vi "Example 2 Primitive Lottery.vi"() -> ()   [LabVIEW 2020]
uses:
  <vilib>/measure/NI_MABase.lvlib
panel:
  out "Fs":dbl format="%#_13g"
  out "Nyquist Eqn":string
  out "cycle of signals":i32
  out "Waveform Graph":waveform(dbl)(graph)
  in  "stop":bool
  in  "amplitude  noise":dbl(knob)=1.0 min=0.001 max=1.0 step=0.1 scale=0.001..1.0
  in  "frequency":dbl(knob)=100.0 min=100.0 max=10000.0 step=10.0 scale=100.0..10000.0
  in  "amplitude":dbl(knob)=1.0 min=0.1 max=10.0 step=0.1 scale=0.1..10.0
  in  "phase":dbl(slide) min=0.0 max=360.0 step=5.0 scale=0.0..360.0
  in  "signal type":T1(ring)
  in  "sampling info":cluster{"Fs":dbl, "#s":dbl}={"Fs"=1000.0, "#s"=1000.0} {"Fs" format="%.2p"}
  in  "square wave duty cycle (%)":dbl=50.0 format="%0.2f"
  in  "offset":dbl(slide)=0.005 min=0.005 max=5.0 step=0.1 scale=0.005..5.0
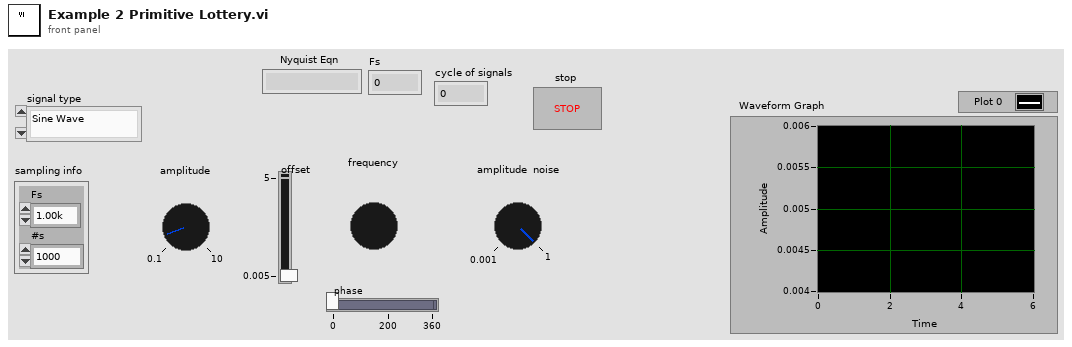
[diagram p1: front panel]
types:
  T1 = enum16{"Sine Wave", "Triangle Wave", "Square Wave", "Sawtooth Wave"}
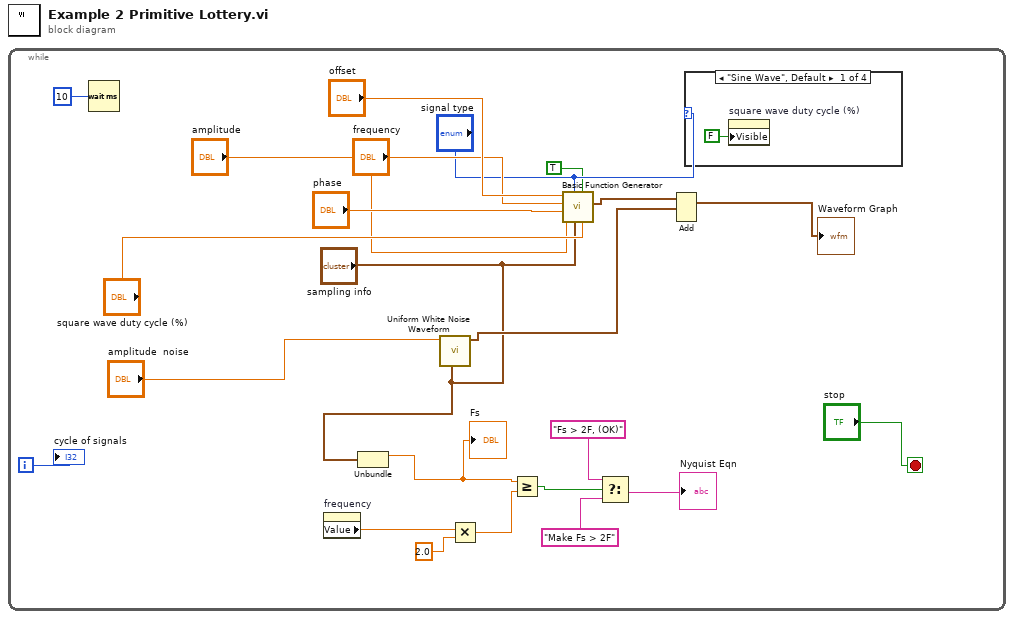
[diagram p0: block diagram]
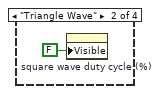
[diagram p2: hidden frame]
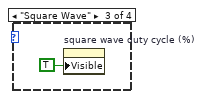
[diagram p3: hidden frame]
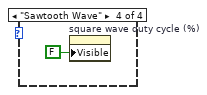
[diagram p4: hidden frame]
diagram:
  n1 = while {
    i -> [w12]
    stop <- "stop" stop-if-true
    n2 = Wait (ms)(milliseconds to wait=10) -> ()  [unwired: 1 out]
    n3 = property on="frequency" class="Knob (strict)"() -> ("Value"=w4:dbl)  [unwired: 2 in, 2 out]
    n4 = Unbundle("sampling info") -> ("Fs"=w2:dbl)  [unwired: 1 out]
    "Fs" <- w2
    n5 = call <vilib>:"Uniform White Noise Waveform.vi"("sampling info"="sampling info", "amplitude"="amplitude  noise") -> ("signal out"=w15:waveform(dbl))  [unwired: 8 in, 1 out]
    n6 = Multiply(x=w4, y=2.0) -> (x*y=w6:dbl)
    n7 = Greater Or Equal?(x=w2, y=w6) -> (x >= y?=w8:bool)
    n8 = call <vilib>:"Basic Function Generator.vi"("offset"="offset", "square wave duty cycle (%)"="square wave duty cycle (%)", "reset signal"=TRUE, "sampling info"="sampling info", "signal type"="signal type", "phase"="phase", "amplitude"="amplitude", "frequency"="frequency") -> ("signal out"=w16:waveform(dbl))  [unwired: 1 in, 2 out]
    n9 = Select(t="Fs > 2F, (OK)", s=w8, f="Make Fs > 2F") -> (s? t:f=→"Nyquist Eqn":string)
    n10 = Add(1:w15, 2:w16) -> (0:→"Waveform Graph":waveform(dbl))  [unwired: 1 in, 1 out]
    n11 = case shown="\"Sine Wave\", Default" "signal type" {
      frame "Sine Wave", Default {
        n12 = property on="square wave duty cycle (%)" class="DigNum (strict)"("Visible"=FALSE) -> ()  [unwired: 2 in, 2 out]
      }
      frame "Triangle Wave" {
        n13 = property on="square wave duty cycle (%)" class="DigNum (strict)"("Visible"=FALSE) -> ()  [unwired: 2 in, 2 out]
      }
      frame "Square Wave" {
        n14 = property on="square wave duty cycle (%)" class="DigNum (strict)"("Visible"=TRUE) -> ()  [unwired: 2 in, 2 out]
      }
      frame "Sawtooth Wave" {
        n15 = property on="square wave duty cycle (%)" class="DigNum (strict)"("Visible"=FALSE) -> ()  [unwired: 2 in, 2 out]
      }
    }
    "cycle of signals" <- w12
  }
